vi "svc_Check for Waveform Parameter Continuity (N Ch).vi"(7 "restart averaging (F)":bool, 8 "error in (no error)":errorcluster, 9 "checks for multichannel parameters":T4, 10 "checks for channel parameter change":T5, 11 "scaled signal(s)":waveform(dbl)[](array[waveform])) -> (0 "error out":errorcluster, 1 "multichannel parameter changed":bool, 2 "waveform parameter changed":bool, 3 "dup scaled signal(s)":waveform(dbl)[](array[waveform]), 4 "array length":i32, 5 "dt":dbl, 6 "channel info":T1[](array[typedef]) {"pregain" format="%.2f"; "weighting filter" items=["Linear", "A-weighting", "B-weighting", "C-weighting", "ITU-R 468-4", "Dolby", "CCITT", "C-message", "Wb", "Wc", "Wd", "We", "Wf", "Wh", "Wj", "Wk", "Wm", "AES17 20 kHz lowpass", "AES17 40 kHz lowpass", "AES17 20 kHz highpass", "AES17 40 kHz highpass"]; "dB reference" format="%^.1e"; "engineering units" items=["custom..."=0, "V"=1, "A"=21, "C"=30, "pC"=31, "s"=32, "-"=29, "Pa"=2, "N"=20, "g"=3, "m/s^2"=4, "m/s"=5, "m"=6, "mm/s"=12, "mm"=13, "micron/s"=14, "micron"=15, "in/s^2"=7, "in/s"=8, "in"=9, "mil/s"=10, "mil"=11, "rad/s^2"=16, "rad/s"=17, "rad"=18, "deg/s^2"=26, "deg/s"=27, "deg"=28, "RPM"=22, "cycle/s^2"=23, "Hz"=24, "cycle"=25, "strain"=19]; "sensor sensitivity" format="%#_5f"})   [LabVIEW 2017]
uses:
  <vilib>/addons/_NISVFA/_Shared subVIs/Controls/svc_Channel Info.ctl
  <vilib>/addons/_NISVFA/_Shared subVIs/Controls/svc_Engineering Units Text Ring.ctl
  <vilib>/addons/_NISVFA/_Shared subVIs/Controls/svc_Weighting Filter Text Ring.ctl
  <vilib>/addons/_NISVFA/_Shared subVIs/Common/svc_Get SV Channel Info.vi
  <vilib>/addons/_NISVFA/_Shared subVIs/Common/svc_Engineering Units to Unit Label.vi
  <vilib>/addons/_NISVFA/_Shared subVIs/Common/svc_Unit Label to Engineering Units.vi
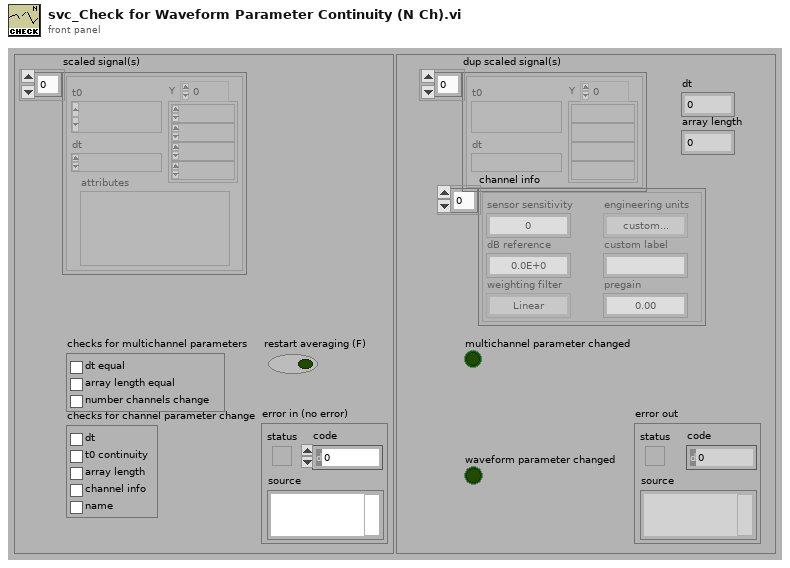
[diagram p1: front panel]
types:
  T1 = typedef "svc_Channel Info.ctl" = cluster{"sensor sensitivity":dbl, "engineering units":T2, "dB reference":dbl, "custom label":string, "weighting filter":T3, "pregain":dbl}
  T2 = typedef "svc_Engineering Units Text Ring.ctl" = u16
  T3 = typedef "svc_Weighting Filter Text Ring.ctl" = u16
  T4 = cluster{"dt equal":bool, "array length equal":bool, "number channels change":bool}
  T5 = cluster{"dt":bool, "t0 continuity":bool, "array length":bool, "channel info":bool, "name":bool}
  T6 = typedef "svc_Waveform Parameters.ctl" = cluster{"channel name":string, "t0":timestamp, "dt":dbl, "array length":i32}
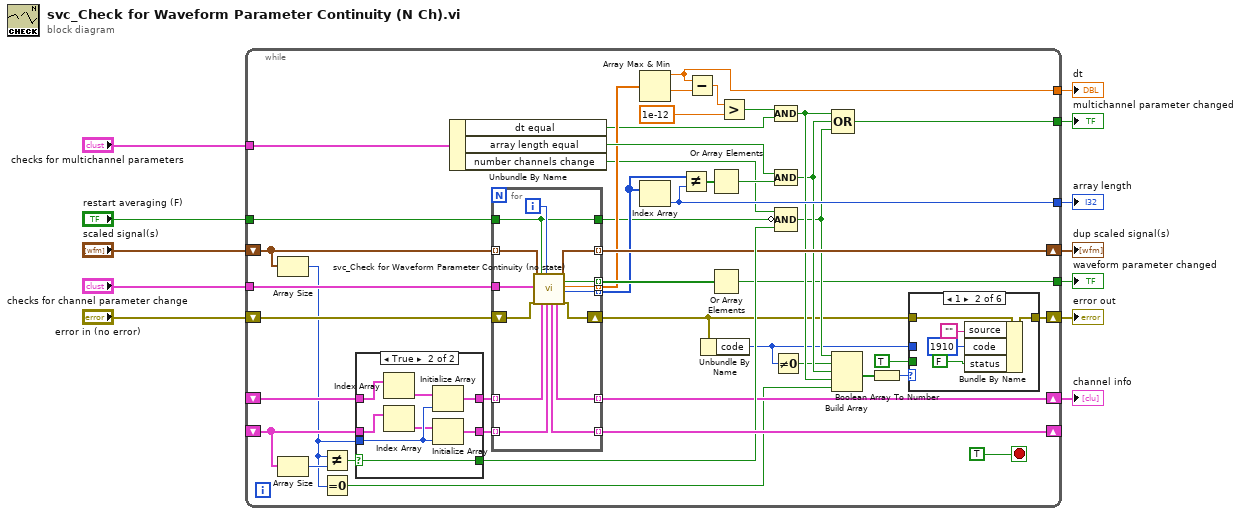
[diagram p0: block diagram]
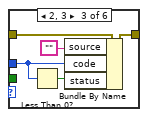
[diagram p3: hidden frame]
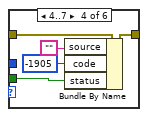
[diagram p4: hidden frame]
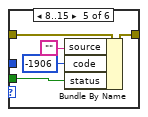
[diagram p5: hidden frame]
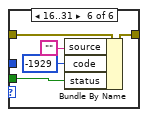
[diagram p6: hidden frame]
diagram:
  n1 = while {
    tunnel: "checks for channel parameter change" -> [w57]
    tunnel: [w20] -> w10
    shift-right: [w55] -> _
    shift-left: _ -> [w52]
    tunnel: "restart averaging (F)" -> [w25]
    tunnel: "checks for multichannel parameters" -> [w39]
    tunnel: [w40] -> w6
    shift-right: [w44] -> w1
    shift-left: _ -> [w43]
    shift-right: [w41] -> w4
    shift-left: "scaled signal(s)" -> [w33]
    tunnel: [w13] -> w3
    tunnel: [w37] -> w2
    shift-right: [w19] -> w12
    shift-left: "error in (no error)" -> [w50]
    stop <- TRUE stop-if-true
    n2 = Array Size(array=w33) -> (size(s)=w32:i32)
    n3 = Array Size(array=w52) -> (size(s)=w54:i32)
    n4 = Not Equal?(x=w32, y=w54) -> (x != y?=w53:bool)
    n5 = Equal To 0?(x=w32) -> (x = 0?=w31:bool)
    n6 = case shown="True" w53 {
      selector: w53 -> [w85 w93]
      tunnel: w52 -> [w86 w91]
      tunnel: [w86 w94] -> w51
      tunnel: w32 -> [_ w92]
      tunnel: [w85 w93] -> w46
      tunnel: [w84 w88] -> w42
      tunnel: w43 -> [w84 w87]
      frame False {
      }
      frame True {
        n7 = Index Array(array=w87) -> (element=w89:T1)  [unwired: 1 in]
        n8 = Index Array(array=w91) -> (element=w90:T6)  [unwired: 1 in]
        n9 = Initialize Array(w89, w92) -> (w88:T1[])
        n10 = Initialize Array(w90, w92) -> (w94:T6[])
      }
    }
    n11 = Unbundle By Name(w39) -> ("dt equal"=w23:bool, "array length equal"=w48:bool, "number channels change"=w26:bool)
    n12 = for {
      tunnel: w57 -> [w102]
      tunnel: w33 -> [w100] mode=indexing
      tunnel: [w108] -> w55 mode=indexing
      tunnel: w51 -> [w107] mode=indexing
      tunnel: w25 -> [w95]
      tunnel: [w99] -> w41 mode=indexing
      tunnel: w42 -> [w97] mode=indexing
      tunnel: [w96] -> w44 mode=indexing
      tunnel: [w103] -> w38 mode=indexing
      tunnel: [w104] -> w35 mode=indexing
      tunnel: [w105] -> w45 mode=indexing
      shift-right: [w106] -> w17
      shift-left: w50 -> [w101]
      tunnel: [w95] -> w16
      i -> [w98]
      n13 = call <vilib>:"svc_Check for Waveform Parameter Continuity (no state).vi"("scaled signal [EU]"=w100, "checks for channel parameter change"=w102, "error in (no error)"=w101, "reset"=w95, "expected channel info"=w97, "channel index"=w98, "expected waveform parameters"=w107) -> ("next expected waveform parameters"=w108:T6, "next expected channel info"=w96:T1, "dup scaled signal [EU]"=w99:waveform(dbl), "waveform parameter changed"=w105:bool, "dt"=w104:dbl, "array length"=w103:i32, "error out"=w106:errorcluster)  [unwired: 6 in]
    }
    n14 = Array Max & Min(array=w35) -> (max value=w13:dbl, min value=w15:dbl)  [unwired: 2 out]
    n15 = Index Array(array=w38) -> (element=w37:i32)  [unwired: 1 in]
    n16 = Not Equal?(x=w38, y=w37) -> (x != y?=w36:bool[])
    n17 = Subtract(x=w13, y=w15) -> (x-y=w34:dbl)
    n18 = Unbundle By Name(w17) -> ("code"=w18:i32)
    n19 = Or Array Elements(Boolean array=w36) -> (logical OR=w47:bool)
    n20 = Or Array Elements(Boolean array=w45) -> (logical OR=w20:bool)
    n21 = Greater?(x=w34, y=1e-12 ("x")) -> (0:w49:bool)
    n22 = Not Equal To 0?(x=w18) -> (x != 0?=w28:bool)
    n23 = Compound Arithmetic op=AND(w49, w23) -> (w30:bool)
    n24 = Compound Arithmetic op=AND(w48, w47) -> (w29:bool)
    n25 = Compound Arithmetic op=AND(w26, invert w16, w46) -> (w27:bool)
    n26 = Compound Arithmetic op=OR(w30, w29, w27) -> (w40:bool)
    n27 = Build Array(w27, w28, w29, w30, w31) -> (w24:bool[])
    n28 = Boolean Array To Number(Boolean array=w24) -> (number=w21:u32)
    n29 = case shown="1" w21 {
      tunnel: w17 -> [w58 w63 w68 w73 w78 w83]
      tunnel: [w58 w62 w67 w72 w77 w82] -> w19
      tunnel: TRUE ("status") -> [_ _ _ w69 w74 w79]
      tunnel: w18 -> [_ _ w64 _ _ _]
      frame 0, Default {
      }
      frame 1 {
        n30 = Bundle By Name(cluster=w63, "source"="", "code"=1910, "status"=FALSE) -> (w62:errorcluster)
      }
      frame 2, 3 {
        n31 = Less Than 0?(x=w64) -> (x < 0?=w65:bool)
        n32 = Bundle By Name(cluster=w68, "source"="", "code"=w64, "status"=w65) -> (w67:errorcluster)
      }
      frame 4..7 {
        n33 = Bundle By Name(cluster=w73, "source"="", "code"=-1905, "status"=w69) -> (w72:errorcluster)
      }
      frame 8..15 {
        n34 = Bundle By Name(cluster=w78, "source"="", "code"=-1906, "status"=w74) -> (w77:errorcluster)
      }
      frame 16..31 {
        n35 = Bundle By Name(cluster=w83, "source"="", "code"=-1929, "status"=w79) -> (w82:errorcluster)
      }
    }
  }
  "error out" <- w12
  "waveform parameter changed" <- w10
  "multichannel parameter changed" <- w6
  "dup scaled signal(s)" <- w4
  "array length" <- w2
  "dt" <- w3
  "channel info" <- w1
